vi "Configure Limit Test.vi"(0 "VISA resource name":refnum<visa-resource-name>, 5 "Limit Line (1)":i32=1 min=1 max=6, 7 "Enable Judge (F:Disable)":bool, 9 "Active Trace (0:A)":i32(ring) items=["A", "B", "C", "D", "E", "F"], 11 "error in (no error)":errorcluster) -> (4 "VISA resource name out":refnum<visa-resource-name>, 15 "error out":errorcluster)   [LabVIEW 2020, in "Anritsu Signal Analyzer Series.lvlib"]
doc: "Configures the limit test settings of the spectrum analyzer."
uses:
  Anritsu Signal Analyzer Series.lvlib
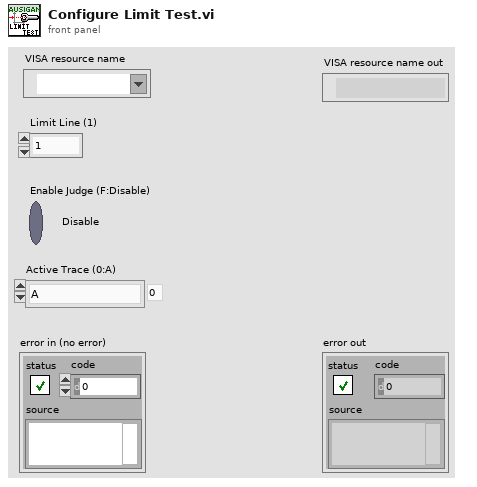
[diagram p1: front panel]
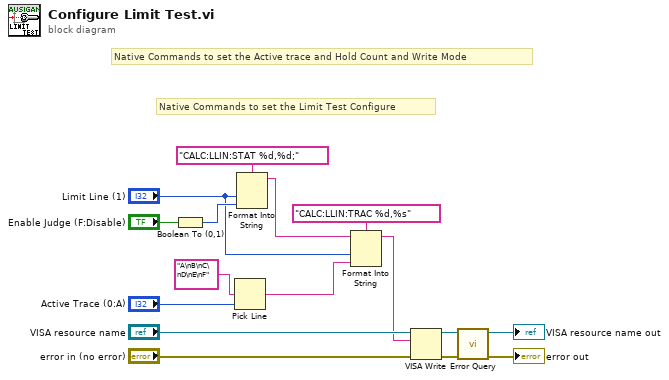
[diagram p0: block diagram]
diagram:
  # "Native Commands to set the Limit Test Configure"
  # "Native Commands to set the Active trace and Hold Count and Write Mode"
  n1 = Boolean To (0,1)(Boolean="Enable Judge (F:Disable)") -> (0, 1=w6:i16)
  n2 = Pick Line(multi-line string="A\nB\nC\nD\nE\nF" ("複数行文字列"), line index="Active Trace (0:A)") -> (output string=w4:string)  [unwired: 1 in]
  n3 = Format Into String(format string="CALC:LLIN:STAT %d,%d;", "Limit Line (1)", w6) -> (resulting string=w2:string)  [unwired: 2 in, 1 out]
  n4 = Format Into String(format string="CALC:LLIN:TRAC %d,%s", initial string=w2, "Limit Line (1)", w4) -> (resulting string=w1:string)  [unwired: 1 in, 1 out]
  n5 = VISA Write(VISA resource name="VISA resource name", write buffer=w1, error in (no error)="error in (no error)") -> (VISA resource name out=w12:refnum<visa-resource-name>, error out=w11:errorcluster)  [unwired: 1 out]
  n6 = call "Error Query.vi"("error in (no error)"=w11, "VISA resource name"=w12) -> ("error out"=→"error out":errorcluster, "VISA resource name out"=→"VISA resource name out":refnum<visa-resource-name>)  [unwired: 6 in, 2 out]
